vi "Write Child Nodes.vi"(8 "error in (no error)":errorcluster, 10 "Child Nodes":map{i64, refnum<class "Messenger.lvclass">}(c390), 11 "Messenger Map Composite in":refnum<class "Messenger Map Composite.lvclass">) -> (0 "error out":errorcluster, 3 "Messenger Map Composite out":refnum<class "Messenger Map Composite.lvclass">)   [LabVIEW 2024, in "Messenger Map Composite.lvclass"]
uses:
  Messenger Map Composite.lvclass
  Messenger/Messenger.lvclass
  Messenger Map Composite.lvclass/Messenger Map Composite.ctl
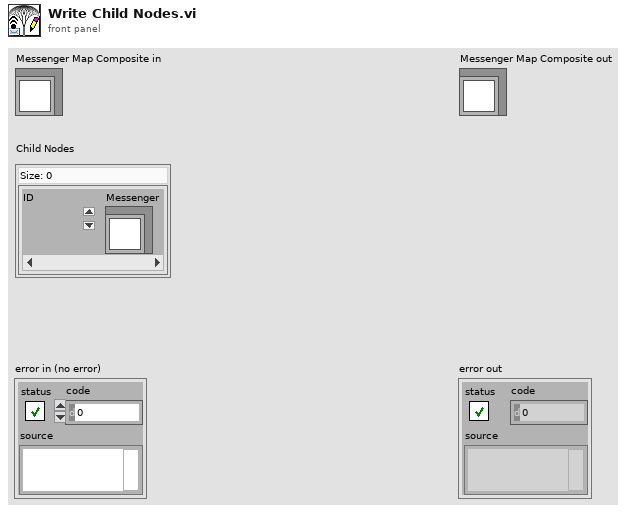
[diagram p1: front panel]
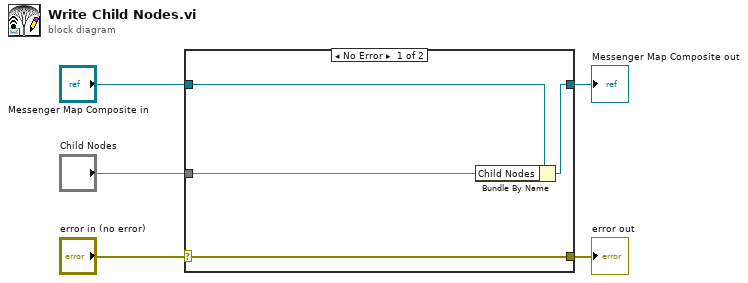
[diagram p0: block diagram]
diagram:
  n1 = case shown="No Error" "error in (no error)" {
    selector: "error in (no error)" -> [w9 w10]
    tunnel: [w9 w10] -> w4
    tunnel: [w7 w11] -> w2
    tunnel: "Messenger Map Composite in" -> [w8 w11]
    tunnel: "Child Nodes" -> [w6 _]
    frame No Error {
      n2 = Bundle By Name(cluster=w8, "Child Nodes"=w6) -> (w7:refnum<class "Messenger Map Composite.lvclass">)
    }
    frame Error {
    }
  }
  "error out" <- w4
  "Messenger Map Composite out" <- w2
